vi "determineClassHierarchy__ogtk.vi"(8 "error in (no error)":errorcluster, 9 "classNames":string[](array[string]), 10 "classObjects":refnum<class>[](array[class])) -> (0 "error out":errorcluster, 2 "hierarchy":string[][](array[string]))   [LabVIEW 2023, in "openg_variant.lvlib" / "Reflection__ogtk.lvclass"]
doc: "Given an array of object and class names, this VI programmatically determines the class hierarchy. The output format is a table, where the first column contains each class name, subsequent columns are descendants of that class.\n\nGCraftsman JSON Object Serialization Toolkit\nwww.GCraftsman.com\nCopyright (c) 2017, GCraftsman"
uses:
  Reflection__ogtk.lvclass
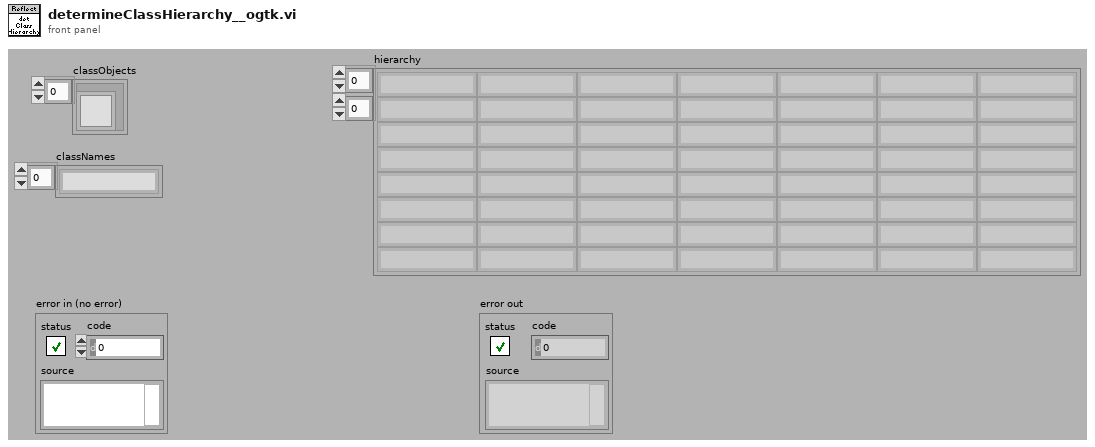
[diagram p1: front panel]
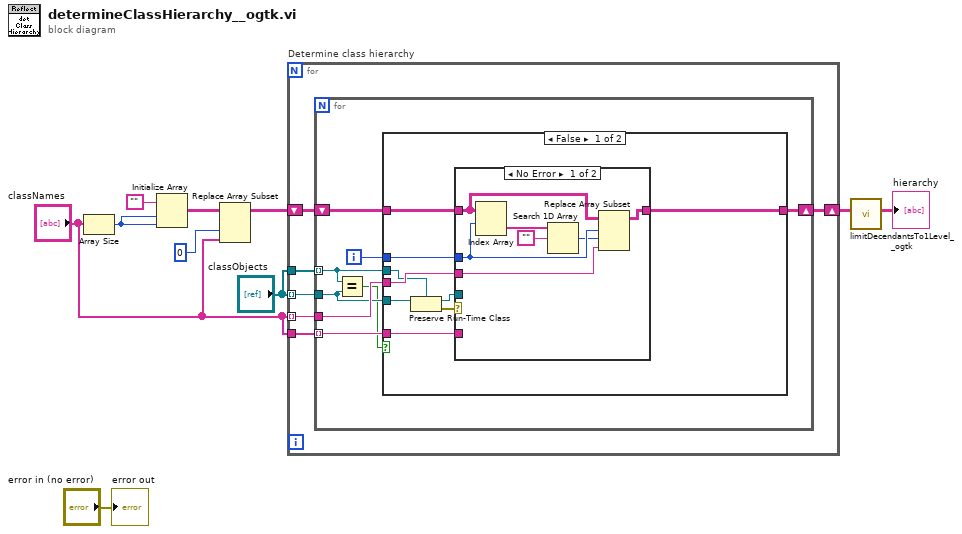
[diagram p0: block diagram]
diagram:
  n1 = Array Size(array="classNames") -> (size(s)=w9:i32)
  n2 = Initialize Array("", w9, w9) -> (w7:string[][])
  n3 = Replace Array Subset(array=w7, new element="classNames", index (col)=0 ("disabled index (col)")) -> (w4:string[][])  [unwired: 1 in]
  n4 = for "Determine class hierarchy" {
    tunnel: "classObjects" -> [w15]
    tunnel: "classObjects" -> [w16] mode=indexing
    tunnel: "classNames" -> [w14] mode=indexing
    tunnel: "classNames" -> [w13]
    shift-right: [w11] -> w3
    shift-left: w4 -> [w12]
    n5 = for {
      tunnel: w16 -> [w21]
      tunnel: w15 -> [w22] mode=indexing
      tunnel: w14 -> [w23]
      tunnel: w13 -> [w24] mode=indexing
      shift-right: [w18] -> w11
      shift-left: w12 -> [w19]
      i -> [w17]
      n6 = Equal?(x=w22, y=w21) -> (x = y?=w20:bool)
      n7 = case shown="False" w20 {
        tunnel: w24 -> [w33 _]
        tunnel: w23 -> [w32 _]
        tunnel: w22 -> [w26 _]
        tunnel: w21 -> [w25 _]
        tunnel: w19 -> [w29 w42]
        tunnel: [w28 w42] -> w18
        tunnel: w17 -> [w27 _]
        frame False {
          n8 = Preserve Run-Time Class(object in=w25, 2:w26) -> (object out=w30:refnum<class>, error out=w31:errorcluster)  [unwired: 1 in]
          n9 = case shown="No Error" w31 {
            tunnel: w32 -> [w34 _]
            tunnel: w33 -> [_ _]
            tunnel: w30 -> [_ _]
            tunnel: w29 -> [w38 w41]
            tunnel: w27 -> [w36 _]
            tunnel: [w37 w41] -> w28
            frame No Error {
              n10 = Index Array(array=w38, index (row)=w36) -> (element=w40:string[])  [unwired: 1 in]
              n11 = Search 1D Array(1D array=w40, element="") -> (index of element=w35:i32)  [unwired: 1 in]
              n12 = Replace Array Subset(array=w38, new element=w34, index (row)=w36, index (col)=w35) -> (w37:string[][])
            }
            frame Error {
            }
          }
        }
        frame True {
          # "skip comparison to self"
        }
      }
    }
  }
  n13 = call "limitDecendantsTo1Level__ogtk.vi"("hierarchy"=w3) -> ("hierarchy out"=→"hierarchy":string[][])  [unwired: 8 in, 2 out]
  "error out" <- "error in (no error)"
